vi "IEPE - Continuous Input - FFT.vi"() -> ()   [LabVIEW 2022 SP3]
doc: "This example demonstrates how to continuously acquire buffered acceleration, sound pressure, or force measurements from IEPE sensors using a DAQmx device.\n\nFor instructions on how to connect your signals to the DAQ device, refer to your device documentation."
uses:
  <vilib>/Utility/error.llb/DialogType.ctl
  <vilib>/DAQmx/read.llb/DAQmx Read (Analog 1D Wfm NChan NSamp).vi
  <vilib>/DAQmx/read.llb/DAQmx Read (Analog Wfm 1Chan NSamp).vi
  <vilib>/DAQmx/create/channels.llb/DAQmx Create Channel (AI-Acceleration-Accelerometer).vi
  <vilib>/DAQmx/create/channels.llb/DAQmx Create Channel (AI-Force-IEPE Sensor).vi
  <vilib>/DAQmx/create/channels.llb/DAQmx Create Channel (AI-Sound Pressure-Microphone).vi
  <vilib>/DAQmx/configure/timing.llb/DAQmx Timing (Sample Clock).vi
  <vilib>/DAQmx/configure/task.llb/DAQmx Configure Logging (TDMS).vi
  <vilib>/DAQmx/configure/trigger.llb/DAQmx Start Trigger (Digital Edge).vi
  <vilib>/DAQmx/configure/trigger.llb/DAQmx Start Trigger (Time).vi
  <vilib>/DAQmx/configure/trigger.llb/DAQmx Start Trigger (Analog Edge).vi
  <vilib>/DAQmx/miscellaneous.llb/DAQmx Fill In Error Info.vi
  <vilib>/measure/maspectr.llb/FFT Spectrum (Mag-Phase) for 1 Chan.vi
  <resource>/objmgr/daqmx.rc
  <vilib>/measure/NI_MAPro.lvlib
panel:
  in  "Window":dbl
  out "Boolean":bool
  in  "Restart Aaveraging":bool
  out "Phase":cluster{"f0":dbl, "df":dbl, "phase":dbl[]}(graph)
  out "Mag":cluster{"f0":dbl, "df":dbl, "magnitude":dbl[]}(graph)
  in  "Trigger Type":T1(tab)
  in  "Digital Start Trigger Edge":i32(ring)=10280 caption="Edge" items=["Rising"=10280, "Falling"=10171]
  in  "Digital Start Trigger Source":tag="/Dev1/PFI0" caption="Source"
  in  "Digital Pause Trigger Pause When":i32(ring)=10192 caption="Pause When" items=["High"=10192, "Low"=10214]
  in  "Digital Pause Trigger Source":tag="/Dev1/PFI0" caption="Source"
  in  "Analog Start Trigger Level":dbl caption="Level" format="%0.2f"
  in  "Analog Start Trigger Hysteresis":dbl caption="Hysteresis" format="%.2f"
  in  "Analog Start Trigger Slope":i32(ring)=10280 caption="Slope" items=["Rising"=10280, "Falling"=10171]
  in  "Analog Start Trigger Source":string="APFI0" caption="Source"
  in  "Analog Pause Trigger Source":string="APFI0" caption="Source"
  in  "Analog Pause Trigger Pause When":i32(ring)=10093 caption="Pause When" items=["Above Level"=10093, "Below Level"=10107]
  in  "Analog Pause Trigger Level":dbl caption="Level" format="%.2f"
  in  "When":timestamp
  in  "Select Time\nManually":bool
  in  "IEPE Current Value (A)":dbl=0.002
  in  "IEPE Excitation Source":i32(ring)=10200 items=["Internal"=10200, "External"=10167, "None"=10230]
  in  "Terminal Configuration":i32(ring)=-1 items=["default"=-1, "RSE"=10083, "NRSE"=10078, "Differential"=10106, "Pseudodifferential"=12529]
  in  "Physical Channel":tag="Dev1/ai0"
  in  "Task Type":T2(tab)
  in  "Min Acceleration":dbl=-100.0
  in  "Max Acceleration":dbl=100.0
  in  "Sensitivity":dbl=95.4
  in  "Acceleration Units":i32(ring)=10186 items=["g"=10186, "m/s^2"=12470, "in/s^2"=12471, "From Custom Scale"=10065]
  in  "Sensitivity Units":i32(ring)=12509 items=["mVolts/ms^2"=0, "mVolts/g"=12509, "Volts/g"=12510]
  in  "Max Sound Pressure Level (dB)":dbl=120.0
  in  "Sound Pressure Units":i32(ring)=10081 items=["Pascals"=10081, "From Custom Scale"=10065]
  in  "Microphone Sensitivity":dbl=10.0
  in  "Sensitivity":dbl=50.0
  in  "Min Force":dbl=-100.0
  in  "Max Force":dbl=100.0
  in  "Sensitivity Units":i32(ring)=15891 items=["mVolts/N"=15891, "mVolts/lb"=15892]
  in  "Force Units":i32(ring)=15875 items=["Newtons"=15875, "Pounds"=15876, "From Custom Scale"=10065]
  in  "Stop":bool
  out "Waveform Graph":waveform(dbl)[](graph)
  in  "TDMS File Path":path
  in  "Samples per Loop":i32=40000
  in  "Sample Rate":dbl=40000.0
  in  "Sample Clock Source":tag="OnboardClock"
  out "Actual Sample Rate":dbl=1000.0000111176631 format="%0.2f"
  in  "Logging Mode":i32(ring)=10231 items=["Off"=10231, "Log and Read"=15842]
  # "Channel Settings"
  # "Acquired Data"
  # "Trigger Settings"
  # "Timing Settings"
  # "Logging Settings"
  # "To enable triggers, select a tab above, and configure the settings.\n\nNot all hardware supports all trigger types. Refer to your device documentation for more information."
  # "This trigger type is not supported in continuous sample timing. \n\nRefer to your device documentation for more information on which triggers are supported."
  # "This trigger type is not supported in continuous sample timing. \n\nRefer to your device documentation for more information on which triggers are supported."
  # "If time is not manually set, task will begin after 10 seconds"
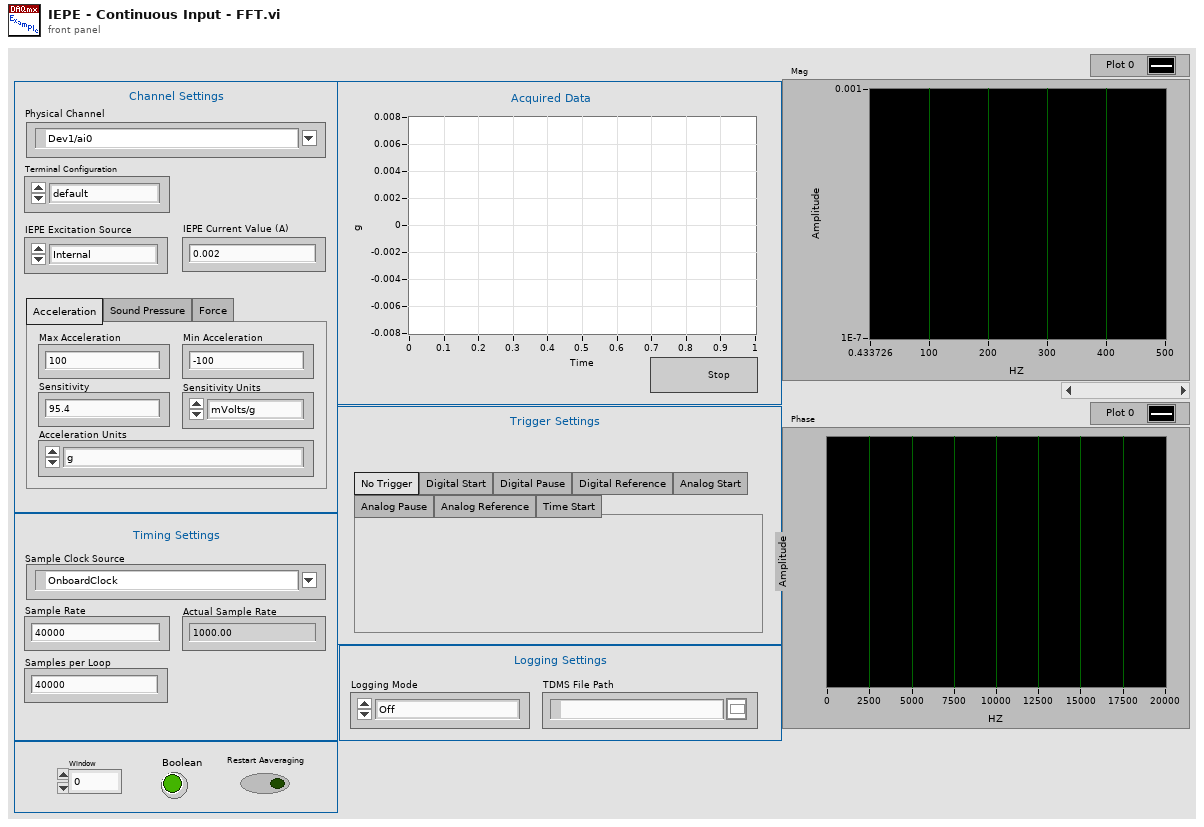
[diagram p1: front panel]
types:
  T1 = enum32{"No Trigger", "Digital Start", "Digital Pause", "Digital Reference", "Analog Start", "Analog Pause", "Analog Reference", "Time Start"}
  T2 = enum32{"Acceleration", "Sound Pressure", "Force"}
  T3 = typedef "DialogType.ctl" = u16
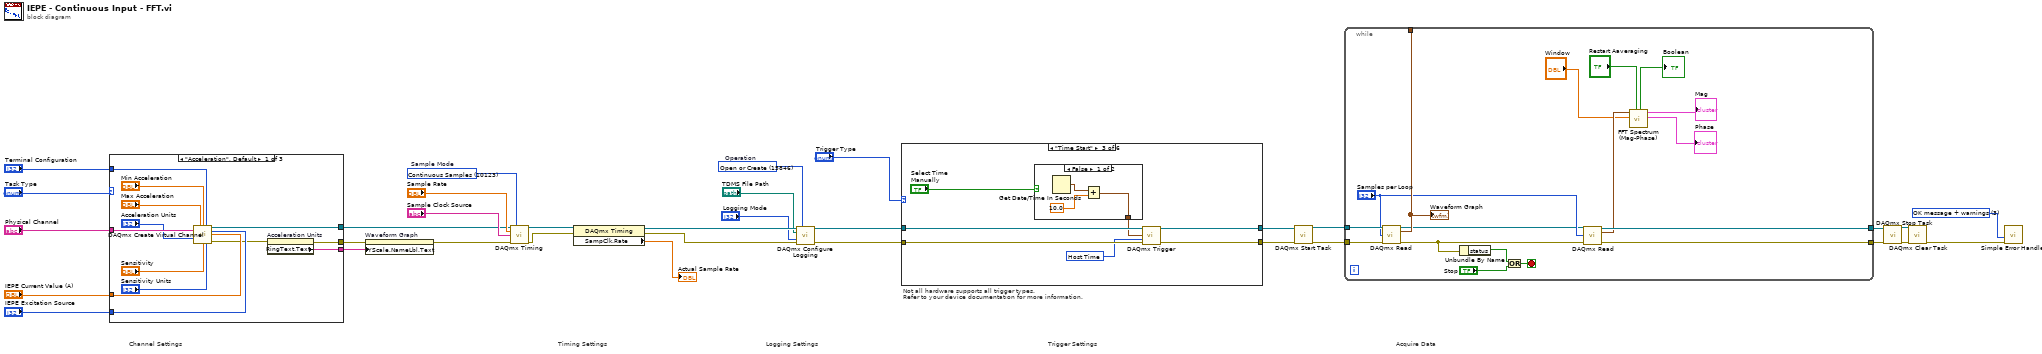
[diagram p0: block diagram]
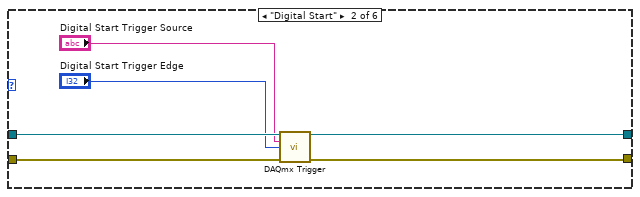
[diagram p3: hidden frame]
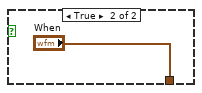
[diagram p4: hidden frame]
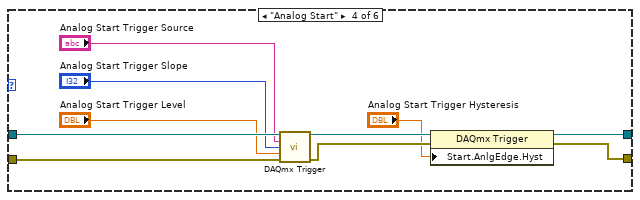
[diagram p5: hidden frame]
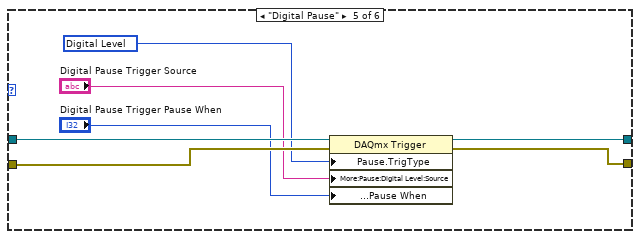
[diagram p6: hidden frame]
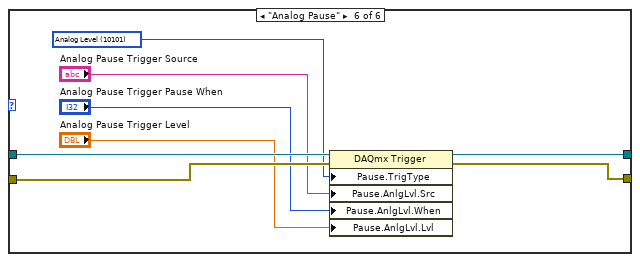
[diagram p7: hidden frame]
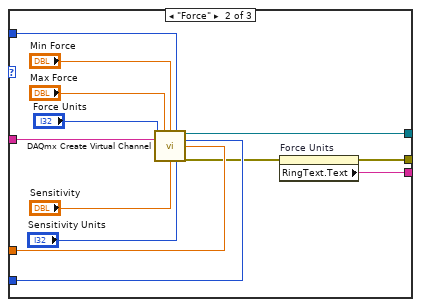
[diagram p8: hidden frame]
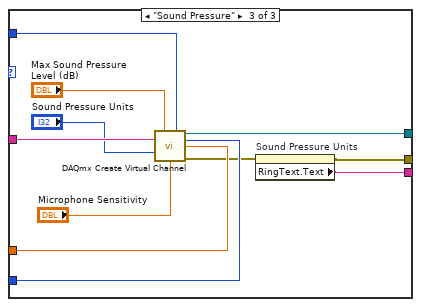
[diagram p9: hidden frame]
diagram:
  w11 = T3 3 items=["no dialog", "OK message", "continue or stop message", "OK message + warnings", "continue/stop + warnings"] ("type of dialog (OK msg:1)")
  w28 = 15846 items=["Open"=10437, "Open or Create"=15846, "Create or Replace"=15847, "Create"=15848]  # Operation
  w31 = 10123 items=["Finite Samples"=10178, "Continuous Samples"=10123, "Hardware Timed Single Point"=12522]  # Sample Mode
  # "Trigger Settings"
  # "Not all hardware supports all trigger types.\nRefer to your device documentation for more information."
  # "Acquire Data"
  # "Timing Settings"
  # "Channel Settings"
  # "Logging Settings"
  n1 = case shown="\"Acceleration\", Default" "Task Type" {
    tunnel: [w36 w49 w63] -> w16
    tunnel: [w46 w59 w70] -> w17
    tunnel: "Physical Channel" -> [w45 w58 w69]
    tunnel: "IEPE Excitation Source" -> [w44 w57 w65]
    tunnel: "IEPE Current Value (A)" -> [w43 w56 w66]
    tunnel: "Terminal Configuration" -> [w42 w55 w68]
    tunnel: [w34 w48 w62] -> w15
    frame "Acceleration", Default {
      n2 = call-poly <vilib>:"DAQmx Create Virtual Channel.vi"("maximum value"="Max Acceleration", "minimum value"="Min Acceleration", "input terminal configuration"=w42, "physical channels"=w45, "current excitation source"=w44, "current excitation value"=w43, "units"="Acceleration Units", "sensitivity"="Sensitivity", "sensitivity units"="Sensitivity Units") -> ("task out"=w46:refnum<k21>, "error out"=w35:errorcluster)  [unwired: 5 in]
      n3 = property on="Acceleration Units" class="Ring (strict)"(error in=w35) -> (error out=w36:errorcluster, "RingText.Text"=w34:string)  [unwired: 1 in, 1 out]
    }
    frame "Force" {
      n4 = call-poly <vilib>:"DAQmx Create Virtual Channel.vi"("maximum value"="Max Force", "minimum value"="Min Force", "input terminal configuration"=w55, "physical channels"=w58, "current excitation source"=w57, "current excitation value"=w56, "units"="Force Units", "sensitivity"="Sensitivity", "sensitivity units"="Sensitivity Units") -> ("task out"=w59:refnum<k21>, "error out"=w47:errorcluster)  [unwired: 5 in]
      n5 = property on="Force Units" class="Ring (strict)"(error in=w47) -> (error out=w49:errorcluster, "RingText.Text"=w48:string)  [unwired: 1 in, 1 out]
    }
    frame "Sound Pressure" {
      n6 = call-poly <vilib>:"DAQmx Create Virtual Channel.vi"("maximum sound pressure level"="Max Sound Pressure Level (dB)", "input terminal configuration"=w68, "physical channels"=w69, "current excitation source"=w65, "current excitation value"=w66, "units"="Sound Pressure Units", "microphone sensitivity"="Microphone Sensitivity") -> ("task out"=w70:refnum<k21>, "error out"=w61:errorcluster)  [unwired: 7 in]
      n7 = property on="Sound Pressure Units" class="Ring (strict)"(error in=w61) -> (error out=w63:errorcluster, "RingText.Text"=w62:string)  [unwired: 1 in, 1 out]
    }
  }
  n8 = property on="Waveform Graph" class="WFGraph (strict)"(error in=w16, "YScale.NameLbl.Text"=w15) -> (error out=w14:errorcluster)  [unwired: 1 in, 1 out]
  n9 = call-poly <vilib>:"DAQmx Timing.vi"("task/channels in"=w17, "sample mode"=w31, "rate"="Sample Rate", "source"="Sample Clock Source", "error in"=w14) -> ("task out"=w33:refnum<k21>, "error out"=w32:errorcluster)  [unwired: 9 in]
  n10 = property class="DAQmx Timing"(reference=w33, error in=w32) -> (reference out=w30:refnum<k21>, error out=w29:errorcluster, "SampClk.Rate"=→"Actual Sample Rate":dbl)
  n11 = call-poly <vilib>:"DAQmx Configure Logging.vi"("task/channels in"=w30, "operation"=w28, "file path"="TDMS File Path", "logging mode"="Logging Mode", "error in"=w29) -> ("task out"=w8:refnum<k21>, "error out"=w9:errorcluster)  [unwired: 9 in]
  n12 = case shown="\"Time Start\"" "Trigger Type" {
    tunnel: w8 -> [w72 w78 w85 w99 w106 w114]
    tunnel: w9 -> [w71 w77 w84 w98 w103 w111]
    tunnel: [w72 w76 w83 w96 w105 w113] -> w6
    tunnel: [w71 w75 w82 w95 w104 w112] -> w7
    frame "No Trigger", Default {
    }
    frame "Digital Start" {
      n13 = call-poly <vilib>:"DAQmx Trigger.vi"("task/channels in"=w78, "source"="Digital Start Trigger Source", "edge"="Digital Start Trigger Edge", "error in"=w77) -> ("task out"=w76:refnum<k21>, "error out"=w75:errorcluster)  [unwired: 10 in]
    }
    frame "Time Start" {
      w79 = 16126 items=["Host Time"=16126, "I/O Device Time"=16127] ("timescale")
      n14 = case shown="False" "Select Time\nManually" {
        tunnel: [w87 "When"] -> w80
        frame False {
          n15 = Get Date/Time In Seconds() -> (seconds since 1Jan1904=w88:timestamp)
          n16 = Add(x=w88, y=10.0) -> (x+y=w87:timestamp)
        }
        frame True {
        }
      }
      n17 = call-poly <vilib>:"DAQmx Trigger.vi"("task/channels in"=w85, "when"=w80, "timescale"=w79, "error in"=w84) -> ("task out"=w83:refnum<k21>, "error out"=w82:errorcluster)  [unwired: 10 in]
    }
    frame "Analog Start" {
      n18 = call-poly <vilib>:"DAQmx Trigger.vi"("task/channels in"=w99, "source"="Analog Start Trigger Source", "slope"="Analog Start Trigger Slope", "level"="Analog Start Trigger Level", "error in"=w98) -> ("task out"=w94:refnum<k21>, "error out"=w93:errorcluster)  [unwired: 9 in]
      n19 = property class="DAQmx Trigger"(reference=w94, error in=w93, "Start.AnlgEdge.Hyst"="Analog Start Trigger Hysteresis") -> (reference out=w96:refnum<k21>, error out=w95:errorcluster)
    }
    frame "Digital Pause" {
      w102 = 10152 items=["Analog Level"=10101, "Analog Window"=10103, "Digital Level"=10152, "Digital Pattern"=10398, "None"=10230] ("Pause.TrigType")
      n20 = property class="DAQmx Trigger"(reference=w106, error in=w103, "Pause.TrigType"=w102, "More:Pause:Digital Level:Source"="Digital Pause Trigger Source", "More:Pause:Digital Level:Pause When"="Digital Pause Trigger Pause When") -> (reference out=w105:refnum<k21>, error out=w104:errorcluster)
    }
    frame "Analog Pause" {
      w110 = 10101 items=["Analog Level"=10101, "Analog Window"=10103, "Digital Level"=10152, "Digital Pattern"=10398, "None"=10230] ("Pause.TrigType")
      n21 = property class="DAQmx Trigger"(reference=w114, error in=w111, "Pause.TrigType"=w110, "Pause.AnlgLvl.Src"="Analog Pause Trigger Source", "Pause.AnlgLvl.When"="Analog Pause Trigger Pause When", "Pause.AnlgLvl.Lvl"="Analog Pause Trigger Level") -> (reference out=w113:refnum<k21>, error out=w112:errorcluster)
    }
  }
  n22 = call <vilib>:"DAQmx Start Task.vi"("task/channels in"=w6, "error in"=w7) -> ("task out"=w4:refnum<k21>, "error out"=w3:errorcluster)  [unwired: 12 in]
  n23 = while {
    tunnel: w4 -> [w131]
    tunnel: w3 -> [w130]
    tunnel: [w126] -> _
    tunnel: [w125] -> w2
    tunnel: [w116] -> w1
    stop <- w115 stop-if-true
    n24 = call-poly <vilib>:"DAQmx Read.vi"("task/channels in"=w131, "number of samples per channel"="Samples per Loop", "error in"=w130) -> ("task out"=w119:refnum<k21>, "data"=w126:waveform(dbl)[], "error out"=w129:errorcluster)  [unwired: 10 in]
    "Waveform Graph" <- w126
    n25 = Unbundle By Name(w129) -> ("status"=w128:bool)
    n26 = Or(x=w128, y="Stop") -> (x .or. y?=w115:bool)
    n27 = call-poly <vilib>:"DAQmx Read.vi"("task/channels in"=w119, "number of samples per channel"="Samples per Loop", "error in"=w129) -> ("task out"=w125:refnum<k21>, "data"=w118:waveform(dbl), "error out"=w116:errorcluster)  [unwired: 10 in]
    n28 = call-poly <vilib>:"FFT Spectrum (Mag-Phase).vi"("restart averaging (F)"="Restart Aaveraging", "window"="Window", "time signal"=w118) -> ("phase"=→"Phase":cluster{"f0":dbl, "df":dbl, "phase":dbl[]}, "magnitude"=→"Mag":cluster{"f0":dbl, "df":dbl, "magnitude":dbl[]}, "averaging done"=→"Boolean":bool)  [unwired: 4 in, 2 out]
  }
  n29 = call <vilib>:"DAQmx Stop Task.vi"("task/channels in"=w2, "error in"=w1) -> ("task out"=w13:refnum<k21>, "error out"=w12:errorcluster)  [unwired: 12 in]
  n30 = call <vilib>:"DAQmx Clear Task.vi"("task in"=w13, "error in"=w12) -> ("error out"=w5:errorcluster)  [unwired: 13 in]
  n31 = call <vilib>:"Simple Error Handler.vi"("type of dialog (OK msg:1)"=w11, "error in (no error)"=w5) -> ()  [unwired: 3 in, 5 out]
